vi "UpdateFiles.vi"(7 "Qbus":refnum<class "Qbus.lvclass">, 8 "error in (no error)":errorcluster, 9 "buffer location":u32, 10 "data group":string, 11 "config":T1) -> (0 "error out":errorcluster, 3 "config":T1)   [LabVIEW 2017, in "McsaDataEventCreator.lvlib"]
uses:
  <vilib>/addons/InsightCM/Devices/Shared/Mcsa/McsaDataEventCreator/McsaDataEventCreator.lvlib
  <vilib>/addons/InsightCM/Devices/Shared/Mcsa/McsaDataEventCreator/controls/config.ctl
  <vilib>/addons/Qbus/Qbus.lvclass
  <vilib>/addons/InsightCM/Devices/Shared/Common/DVRBuffer/controls/BufferLocation.ctl
  <vilib>/addons/InsightCM/Devices/Shared/Mcsa/McsaDataEventCreator/controls/DataGroupRegistry.ctl
  <vilib>/addons/InsightCM/Devices/Shared/Mcsa/McsaDataEventCreator/controls/Registry_DataSet.ctl
  <vilib>/addons/InsightCM/Devices/Shared/Mcsa/McsaDataEventCreator/controls/DataSetType.ctl
  <vilib>/addons/InsightCM/Devices/Shared/Common/DataEventCreator/controls/Registry_Trend.ctl
  <vilib>/addons/InsightCM/Devices/Shared/Common/DataFlow/controls/Data.ctl
  <vilib>/addons/InsightCM/Utilities/DataAccessors/controls/wfmSGL_DVR.ctl
  <vilib>/addons/PointValueMap/controls/PointMap.ctl
  <vilib>/addons/InsightCM/Devices/Shared/Common/DataFlow/controls/Type.ctl
  <vilib>/addons/InsightCM/Devices/Shared/Common/FileFlow/subVIs/GetFirstProcessModule_EventRef.vi
  <vilib>/addons/InsightCM/Devices/Shared/Common/DVRBuffer/DVRBuffer.lvlib
  <vilib>/addons/PointValueMap/PointValueMap.lvlib
  <vilib>/addons/InsightCM/Devices/Shared/Common/FileFlow/FileFlow.lvlib
  <vilib>/addons/InsightCM/Devices/Shared/Common/DataEventCreator/DataEventCreator.lvlib
  <vilib>/addons/InsightCM/Devices/Shared/Common/DataFlow/DataFlow.lvlib
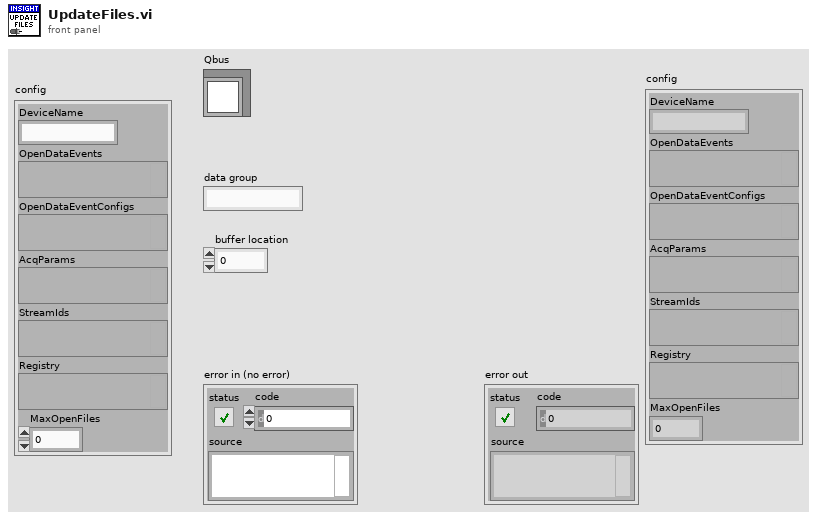
[diagram p1: front panel]
types:
  T1 = typedef "McsaDataEventCreator.lvlib/config.ctl" = cluster{"DeviceName":string, "OpenDataEvents":variant, "OpenDataEventConfigs":variant, "AcqParams":variant, "StreamIds":variant, "Registry":variant, "MaxOpenFiles":i32}
  T2 = typedef "McsaDataEventCreator.lvlib/DataGroupRegistry.ctl" = cluster{"AssetNodeMap":variant, "DataSets":T3[], "Trends":T5[]}
  T3 = typedef "McsaDataEventCreator.lvlib/Registry_DataSet.ctl" = cluster{"ChannelName":string, "DataSetType":T4, "DoNotWriteToDB":bool, "ParentName":string}
  T4 = typedef "McsaDataEventCreator.lvlib/DataSetType.ctl" = enum16{"Waveform", "MCSAFFT", "TorqueWFM"}
  T5 = typedef "DataEventCreator.lvlib/Registry_Trend.ctl" = cluster{"TrendPointId":string, "DataSetName":string, "HighRate":bool, "Always Send":bool}
  T6 = typedef "DVRBuffer.lvlib/BufferLocation.ctl" = cluster{"Block":u32, "Index":i32}
  T7 = typedef "McsaDataEventCreator.lvlib/DataEventConfig.ctl" = cluster{"AcqParams":T8, "OpState":string, "ExitOpState":bool, "Reason":string, "StreamId":string, "Map":T11, "DataSetIds":variant, "IncludeWaveforms":bool, "TrendPointsOnly":bool}
  T8 = typedef "McsaDataEventCreator.lvlib/AcqParams.ctl" = cluster{"Stream":bool, "PreTrigger":i32, "CollectOnEnter":bool, "Enter PreTrigger":i32, "Enter Length":dbl, "CollectOnExit":bool, "ContinuousData":bool, "Accumulation Settings":T9}
  T9 = typedef "DataAccumulator.lvlib/AccumulationSettings.ctl" = cluster{"Type":T10, "Length":dbl, "Max Time (sec)":dbl, "Start Block":T6, "Acquired (sec)":dbl, "Acquired (pulses)":i32, "Initial Pulse Offset":dbl, "Stop Block":T6, "LastBlockAdded":u32}
  T10 = typedef "DataAccumulator.lvlib/accumulationType.ctl" = enum16{"none", "seconds", "revolutions"}
  T11 = typedef "PointValueMap.lvlib/PointMap.ctl" = refnum<data-value>
  T12 = typedef "DataEvent.lvlib/Event.ctl" = cluster{"DataEvent":T13, "DataSets":T15[], "TrendPoints":T17[], "Alarms":T18[]}
  T13 = typedef "DataEvent.ctl" = cluster{"Id":string, "AssetNodeId":string, "Timestamp":i64, "Props":T14[]}
  T14 = typedef "KeyValuePair.ctl" = cluster{"Key":string, "Value":string}
  T15 = typedef "DataEvent.lvlib/DataSet.ctl" = cluster{"DataSetMetadata":T16, "Values":sgl[], "Values DVR":refnum<data-value>}
  T16 = typedef "DataSetMetadata.ctl" = cluster{"Id":string, "DataEventId":string, "AssetNodeId":string, "Type":string, "T0":i64, "Props":T14[]}
  T17 = typedef "TrendPoint.ctl" = cluster{"TrendPointId":string, "DataEventId":string, "Timestamp":i64, "Value":dbl, "Props":T14[]}
  T18 = typedef "TrendAlarmUpdate.ctl" = cluster{"RuleId":string, "Transition":T19}
  T19 = typedef "TrendAlarmTransition.ctl" = cluster{"At":i64, "Severity":i32, "Value":dbl, "Properties":T14[]}
  T20 = typedef "DataFlow.lvlib/Type.ctl" = enum16{"High Rate", "Low Rate", "Burst Mode"}
  T21 = typedef "DataFlow.lvlib/Data.ctl" = cluster{"DataGroup":string, "Waveforms":T22, "Map":T11, "Type":T20}
  T22 = typedef "wfmSGL_DVR.ctl" = refnum<data-value>
  T23 = typedef "FileFlow.lvlib/data_eventRef.ctl" = cluster{"event reference":T24, "DataGroup":string, "OperatingState":string, "StreamId":string, "LastBlock":bool, "Map":T11, "TrendPoints Only":bool, "Extra Large File":bool}
  T24 = typedef "DataEvent.lvlib/EventReference.ctl" = refnum<data-value>
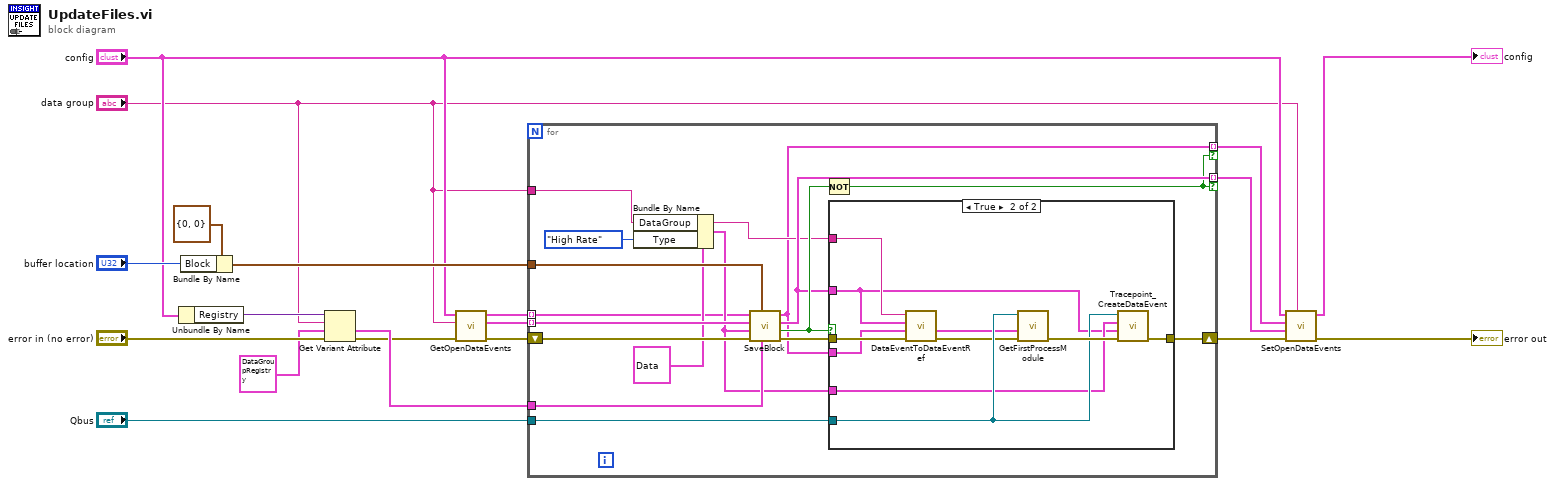
[diagram p0: block diagram]
diagram:
  n1 = Unbundle By Name("config") -> ("Registry"=w17:variant)
  n2 = Bundle By Name(cluster=T6 {"Block"=0, "Index"=0} ("start block"), "Block"="buffer location") -> (w14:T6)
  n3 = Get Variant Attribute(Variant=w17, name="data group", default value (empty Variant)=T2 {"AssetNodeMap"=variant, "DataSets"=[], "Trends"=[]} ("Data Group Registry"), error in="error in (no error)") -> (value=w13:T2, error out=w11:errorcluster)  [unwired: 2 out]
  n4 = call <vilib>:"GetOpenDataEvents.vi"("error in (no error)"=w11, "data group"="data group", "config"="config") -> ("error out"=w10:errorcluster, "open data event configs"=w9:T7[], "open data events"=w8:T12[])  [unwired: 6 in]
  n5 = for {
    tunnel: w9 -> [w28] mode=indexing
    tunnel: "data group" -> [w25]
    tunnel: "Qbus" -> [w31]
    shift-right: [w34] -> w6
    shift-left: w10 -> [w33]
    tunnel: [w29] -> w2 mode=indexing if=w21
    tunnel: w13 -> [w27]
    tunnel: w14 -> [w30]
    tunnel: w8 -> [w23] mode=indexing
    tunnel: [w22] -> w1 mode=indexing if=w21
    n6 = Bundle By Name(cluster=T21 {"DataGroup"="", "Waveforms"=refnum, "Map"=refnum, "Type"=enum."High Rate"} ("data"), "DataGroup"=w25, "Type"=Type."High Rate") -> (w24:T21)
    n7 = call <vilib>:"SaveBlock.vi"("Registry"=w27, "start block"=w30, "error in (no error)"=w33, "data"=w24, "data event config in"=w28, "data event"=w23) -> ("error out"=w35:errorcluster, "file complete"=w32:bool, "data event config out"=w29:T7, "data event out"=w22:T12)  [unwired: 2 in]
    n8 = Not(x=w32) -> (.not. x?=w21:bool)
    n9 = case shown="True" w32 {
      tunnel: w35 -> [w36 w42]
      tunnel: w29 -> [_ w38]
      tunnel: w25 -> [_ w39]
      tunnel: w31 -> [_ w44]
      tunnel: [w36 w45] -> w34
      tunnel: w24 -> [_ w43]
      tunnel: w22 -> [_ w37]
      frame False {
      }
      frame True {
        n10 = call <vilib>:"DataEventToDataEventRef.vi"("error in (no error)"=w42, "data event"=w37, "data event config"=w38, "data group"=w39) -> ("error out"=w41:errorcluster, "data event ref"=w40:T23)  [unwired: 6 in]
        n11 = call-poly <vilib>:"GetFirstProcessModule.vi"("error in (no error)"=w41, "data"=w40, "Qbus in"=w44) -> ("error out"=w46:errorcluster)  [unwired: 7 in, 1 out]
        n12 = call <vilib>:"Tracepoint_CreateDataEvent.vi"("error in (no error)"=w46, "data event"=w38, "data"=w43, "Qbus"=w44) -> ("error out"=w45:errorcluster)  [unwired: 7 in]
      }
    }
  }
  n13 = call <vilib>:"SetOpenDataEvents.vi"("data group"="data group", "error in (no error)"=w6, "data event configs"=w2, "data events"=w1, "config"="config") -> ("error out"=→"error out":errorcluster, "config out"=→"config":T1)  [unwired: 5 in]
